vi "AO Start.vi"(0 "taskID in":u32 format="%x", 5 "number of buffer iterations (1)":i32=1, 7 "update rate (1000 updates/sec)":sgl=1000.0 format="%0.2f", 11 "error in (no error)":errorcluster, 12 "clock (update clock 1:1)":T1(ring), 13 "clock source (internal:1)":u16(ring)=1 items=["no change", "internal", "counter 1", "counter 2", "counter 3", "counter 5", "I/O connector", "RTSI connection", "PFI pin, low to high", "PFI pin, high to low", "RTSI pin, low to high", "RTSI pin, high to low", "GPCTR 1 output, low to high", "GPCTR 1 output, high to low", "ATCOUT, low to high", "ACTOUT, high to low", "internal clock 2"]) -> (4 "taskID out":u32 format="%x", 6 "actual update rate":sgl format="%0.2f", 15 "error out":errorcluster)   [LabVIEW 2009]
doc: "Starts a buffered analog output operation. This VI sets the update rate and then starts the generation."
panel:
  out "task ID out":u32 format="%x"
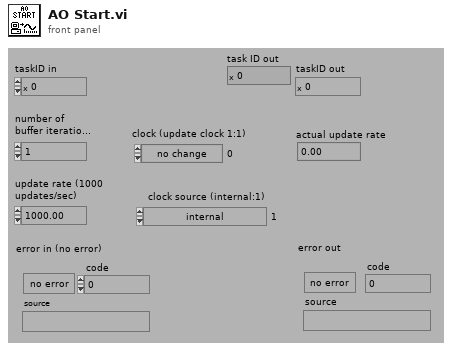
[diagram p1: front panel]
types:
  T1 = enum16{"no change", "update clock 1", "interval clock 1", "update clock 2"}
  T2 = enum16{"start", "pause", "pause at EOC", "resume", "clear", "switch to next buffer", "switch to next buffer at EOC"}
  T3 = cluster{"ticks per second used":sgl, "seconds per tick used":sgl, "timebase signal used":sgl, "timebase divisor used":i32}
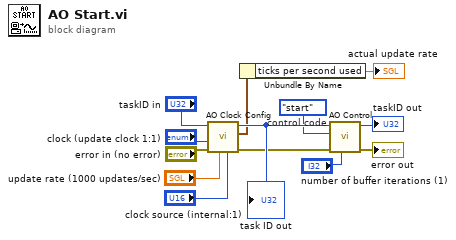
[diagram p0: block diagram]
diagram:
  w2 = T2."start"  # control code
  n1 = call <vilib>:"AO Clock Config.vi"("clock source (0: no change)"="clock source (internal:1)", "ticks per second (-1: no change)"="update rate (1000 updates/sec)", "error in (no error)"="error in (no error)", "clock (0: no change)"="clock (update clock 1:1)", "task ID"="taskID in") -> ("error out"=w8:errorcluster, "actual rates used"=w4:T3, "task ID out"=w9:u32)  [unwired: 4 in]
  "task ID out" <- w9
  n2 = Unbundle By Name(w4) -> ("ticks per second used"=→"actual update rate":sgl)
  n3 = call "AO Control.vi"("iterations (0: infinite)"="number of buffer iterations (1)", "error in (no error)"=w8, "control code (0: start)"=w2, "task ID"=w9) -> ("error out"=→"error out":errorcluster, "task ID out"=→"taskID out":u32)  [unwired: 6 in]
